vi "FPGA VI.vi"() -> ()   [LabVIEW 2026]
uses:
  <vilib>/rvi/Emulation/niFpgaGetClockAttributes.vi
  <vilib>/rvi/Emulation/niFpgaSctlEmulationGetInTimedLoop.vi
  <vilib>/rvi/Emulation/niFpgaEmulationReportErrorSimple.vi
  <vilib>/rvi/Emulation/niFpgaEmulationIsFPGAContextNoSignature.vi
  <vilib>/rvi/errors/niFpgaSetErrorForExecOnDevCompSimple.vi
  <vilib>/rvi/eio/common/nirviEmuReportErrorAndStop.vi
  <vilib>/rvi/DataTransferAndStorage/Container/Common/niFpgaContainerGetUniqueNameForEmu.vi
  <vilib>/rvi/FIFO/Fifo_Resource/nirvififoEmulationSetSize.vi
  <vilib>/rvi/FIFO/Fifo_Resource/nirviFifoEmulationQueueMgr.vi
  <instcachedir>/0/nirviFifoEmulationQueueMgr_E5CAEC123FF24DC58D834DCA3CDAA9B5.lvgen/nirviFifoEmulationQueueMgr_E5CAEC123FF24DC58D834DCA3CDAA9B5_002.vi
  <vilib>/Utility/error.llb/Clear Errors.vi
  <vilib>/rvi/FIFO/Fifo_Resource/nirvififoEmulationCreateLock.vi
  <vilib>/rvi/Emulation/niFpgaProcessEmulError.vi
  <vilib>/rvi/FIFO/Fifo_Resource/nirvififoEmulationObtainLock.vi
  <vilib>/rvi/FIFO/Fifo_Resource/nirvififoEmulationReleaseLock.vi
  <vilib>/rvi/occurrence/nirviWaitOnOccurrenceBase.vi
  <vilib>/rvi/errors/nirviReportUnexpectedCaseInternalError.vi
  <vilib>/rvi/errors/nirviReportUnexpectedCaseInternalError (U32).vi
  <vilib>/rvi/Emulation/niFpgaCriticalErrorInLSC.vi
  <vilib>/rvi/eio/common/nirviEmuTemplateMethod_errors.vi
  <vilib>/rvi/FIFO/Fifo_Resource/nirvififoEmulationDetermineInputValidOut.vi
  <vilib>/rvi/DataTransferAndStorage/Container/XNode/niFpgaContainer.xnode
  <vilib>/rvi/FIFO/Fifo_Resource/nirvififoEmulationRead.vi
  <vilib>/eio/EIONode/EIONode.xnode
  <vilib>/rvi/FIFO/Fifo_Resource/nirvififoEmulationWrite.vi
panel:
  out "appended array 3":bool[](array[boolean])
  out "appended array 2":bool[](array[boolean])
  out "appended array":bool[](array[boolean])
  in  "beep duration":i32=50
  in  "# of LED's lit at once":i16=11
  in  "activation threshold":u32=300
  out "Numeric":i32
  out "Time Since Last":u32=112
  in  "PWM Speaker Freq":u16[](array[numeric])=[432, 543, 754, 865, 1087]
  out "Iteratino Count":i32=5816678
  out "Time Left (ms)":i32
  in  "Random Index":i16
  out "Score":u16=718
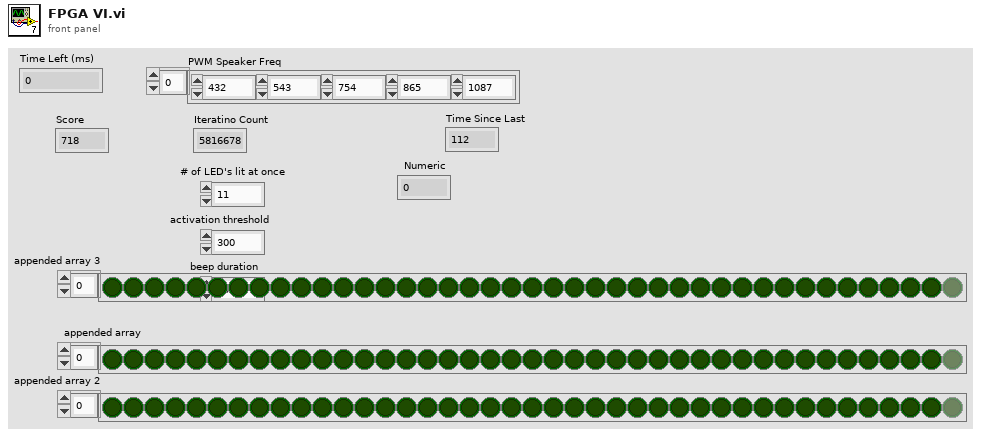
[diagram p1: front panel]
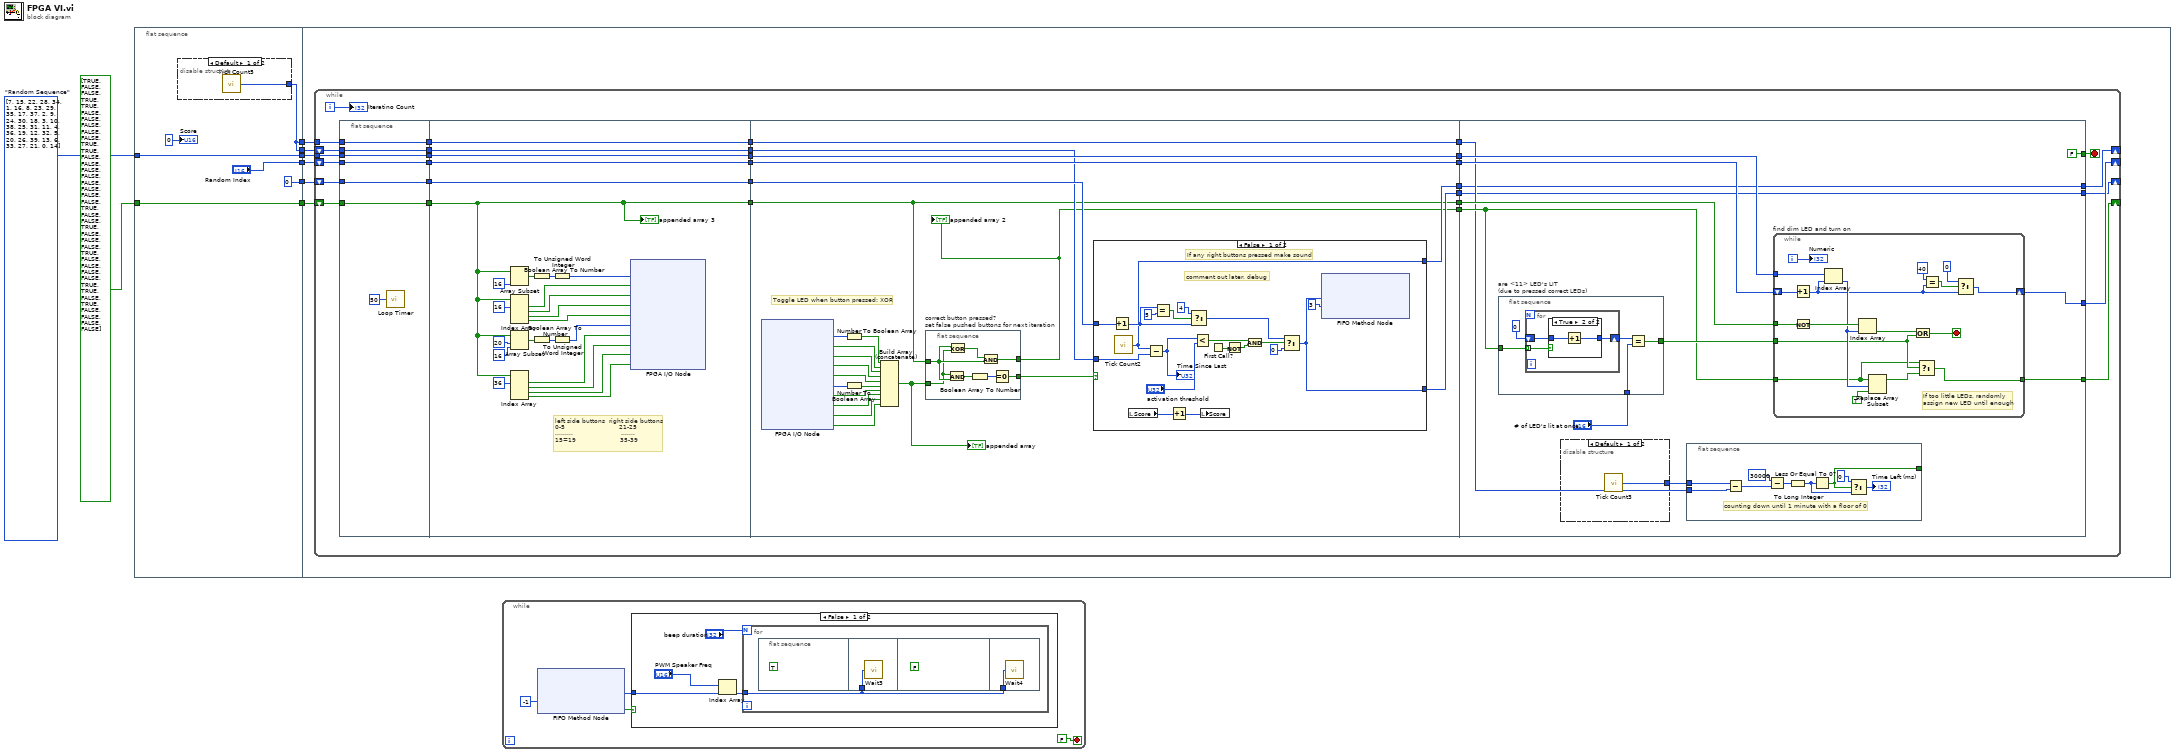
[diagram p0: block diagram]
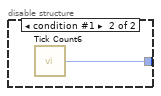
[diagram p3: hidden frame]
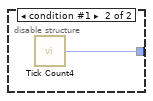
[diagram p5: hidden frame]
diagram:
  w2 = i16[] [7, 15, 22, 28, 34, 1, 16, 8, 23, 29, 35, 17, 37, 2, 9, 24, 30, 18, 3, 10, 38, 25, 31, 11, 4, 36, 19, 12, 32, 5, 20, 26, 39, 13, 6, 33, 27, 21, 0, 14]  # "Random Sequence"
  n1 = flat-sequence {
    tunnel: [w11] -> w8
    tunnel: [w10] -> w7
    tunnel: [w12] -> w6
    tunnel: ["Random Index"] -> w5
    tunnel: [u32 0 ("index")] -> w4
    tunnel: [w11] -> w3
    tunnel: w2 -> [w12]
    tunnel: bool[] [TRUE, FALSE, FALSE, TRUE, TRUE, FALSE, FALSE, FALSE, FALSE, FALSE, TRUE, TRUE, FALSE, FALSE, FALSE, FALSE, FALSE, FALSE, FALSE, FALSE, TRUE, FALSE, FALSE, TRUE, FALSE, FALSE, FALSE, TRUE, FALSE, FALSE, FALSE, FALSE, TRUE, TRUE, FALSE, TRUE, FALSE, FALSE, FALSE, FALSE] ("LEDs lit") -> [w10]
    tunnel: w8 -> [w19]
    tunnel: w7 -> [w22]
    tunnel: w6 -> [w21]
    tunnel: w5 -> [w20]
    tunnel: w4 -> [w18]
    tunnel: w3 -> [w17]
    frame #0 {
      n2 = disable-structure shown="Default" {
        disable-tunnel: [w15 w16] -> w11
        frame condition #0 (active) {
          n3 = call "Tick Count5"() -> ("Tick Count(mSec)"=w15:u32)
        }
        frame condition #1 {
          n4 = call "Tick Count6"() -> ("Tick Count(uSec)"=w16:u32)
        }
      }
      "Score" <- u16 0 ("Score 2")
    }
    frame #1 {
      n5 = while {
        shift-right: [w49] -> _
        shift-left: w22 -> [w52]
        tunnel: w21 -> [w45]
        shift-right: [w39] -> _
        shift-left: w20 -> [w41]
        tunnel: w19 -> [w35]
        shift-right: [w28] -> _
        shift-left: w18 -> [w30]
        shift-right: [w24] -> _
        shift-left: w17 -> [w25]
        i -> [w33]
        stop <- w34 stop-if-true
        n6 = flat-sequence {
          tunnel: [w59] -> w53
          tunnel: w52 -> [w59]
          tunnel: [w58] -> w46
          tunnel: w45 -> [w58]
          tunnel: [w57] -> w42
          tunnel: w41 -> [w57]
          tunnel: [w56] -> w36
          tunnel: w35 -> [w56]
          tunnel: [w55] -> w31
          tunnel: w30 -> [w55]
          tunnel: [w54] -> w26
          tunnel: w25 -> [w54]
          tunnel: w53 -> [w61]
          tunnel: [w61] -> w51
          tunnel: [w85] -> w47
          tunnel: w46 -> [w85]
          tunnel: [w84] -> w43
          tunnel: w42 -> [w84]
          tunnel: [w83] -> w37
          tunnel: w36 -> [w83]
          tunnel: [w82] -> w32
          tunnel: w31 -> [w82]
          tunnel: [w81] -> w27
          tunnel: w26 -> [w81]
          tunnel: w51 -> [w88]
          tunnel: [w86] -> w50
          tunnel: [w107] -> w48
          tunnel: w47 -> [w107]
          tunnel: [w106] -> w44
          tunnel: w43 -> [w106]
          tunnel: [w88] -> w40
          tunnel: [w105] -> w38
          tunnel: w37 -> [w105]
          tunnel: w32 -> [w104]
          tunnel: [w103] -> w29
          tunnel: w27 -> [w102]
          tunnel: [w101] -> w23
          tunnel: w50 -> [w147]
          tunnel: [w148] -> w49
          tunnel: w48 -> [w146]
          tunnel: w44 -> [w145]
          tunnel: w40 -> [w144]
          tunnel: [w143] -> w39
          tunnel: w38 -> [w142]
          tunnel: [FALSE] -> w34
          tunnel: w29 -> [w141]
          tunnel: [w141] -> w28
          tunnel: [w140] -> w24
          tunnel: w23 -> [w140]
          frame #0 {
            n7 = call "Loop Timer"("Count(uSec)"=u8 50 ("Count(Ticks)")) -> ()  [unwired: 1 out]
          }
          frame #1 {
            # "left side buttons  right side buttons\n0-5                           21-25\n.........                        .......  \n15=19                      35-39"
            n8 = Array Subset(array=w61, length=16) -> (w79:bool[])  [unwired: 1 in]
            n9 = Index Array(array=w61, index #1=16 ("index")) -> (element #1=w62:bool, element #2=w65:bool, element #3=w64:bool, element #4=w63:bool)  [unwired: 3 in]
            n10 = Array Subset(array=w61, index=20, length=16) -> (w74:bool[])
            n11 = Index Array(array=w61, index #1=36 ("index")) -> (element #1=w70:bool, element #2=w68:bool, element #3=w67:bool, element #4=w66:bool)  [unwired: 3 in]
            n12 = Boolean Array To Number(Boolean array=w79) -> (number=w78:u16)
            n13 = Boolean Array To Number(Boolean array=w74) -> (number=w75:u16)
            n14 = To Unsigned Word Integer(number=w78) -> (unsigned 16bit integer=w77:u16)
            n15 = To Unsigned Word Integer(number=w75) -> (unsigned 16bit integer=w69:u16)
            n16 = xnode "FPGA I/O Node"("Bank-01/DO15:0"=w77, "Bank-03/DO0"=w62, "Bank-03/DO1"=w65, "Bank-03/DO2"=w64, "Bank-03/DO3"=w63, "Bank-02/DO15:0"=w69, "Bank-03/DO4"=w70, "Bank-03/DO5"=w68, "Bank-03/DO6"=w67, "Bank-03/DO7"=w66) -> ()  [unwired: 10 in, 10 out]
            "appended array 3" <- w61
          }
          frame #2 {
            # "Toggle LED when button pressed: XOR"
            n17 = xnode "FPGA I/O Node"() -> ("Bank-01/DI15:0"=w108:u16, "Bank-03/DI0"=w90:bool, "Bank-03/DI1"=w99:bool, "Bank-03/DI2"=w98:bool, "Bank-03/DI3"=w97:bool, "Bank-02/DI15:0"=w92:u16, "Bank-03/DI4"=w96:bool, "Bank-03/DI5"=w95:bool, "Bank-03/DI6"=w94:bool, "Bank-03/DI7"=w93:bool)  [unwired: 10 in, 10 out]
            n18 = Number To Boolean Array(number=w108) -> (Boolean array=w100:bool[])
            n19 = Number To Boolean Array(number=w92) -> (Boolean array=w91:bool[])
            n20 = Build Array (concatenate)(w100, w90, w99, w98, w97, w91, w96, w95, w94, w93) -> (w87:bool[])
            "appended array" <- w87
            n21 = flat-sequence "correct button pressed?\nset false pushed buttons for next iteration" {
              tunnel: [w114] -> w86
              tunnel: [w111] -> w89
              tunnel: w88 -> [w110]
              tunnel: w87 -> [w109]
              frame #0 {
                n22 = And(x=w109, y=w110) -> (x .and. y?=w113:bool[])
                n23 = Exclusive Or(1:w109, 2:w110) -> (0:w115:bool[])
                n24 = Boolean Array To Number(Boolean array=w113) -> (number=w112:u64)
                n25 = And(x=w115, y=w110) -> (x .and. y?=w114:bool[])
                n26 = Equal To 0?(x=w112) -> (x = 0?=w111:bool)
              }
            }
            n27 = case shown="False" w89 {
              tunnel: w104 -> [w125 w136]
              tunnel: [w116 w136] -> w103
              tunnel: w102 -> [w118 w135]
              tunnel: [w117 w135] -> w101
              frame False {
                # "comment out later, debug"
                # "If any right buttons pressed make sound"
                n28 = Increment(x=w125) -> (x+1=w128:u32)
                n29 = call "Tick Count2"() -> ("Tick Count(mSec)"=w117:u32)
                n30 = local read "Score"() -> (w134:u16)
                n31 = Subtract(x=w117, y=w118) -> (x-y=w119:u32)
                "Time Since Last" <- w119
                n32 = Equal?(x=w128, y=u32 5) -> (x = y?=w130:bool)
                n33 = Increment(x=w134) -> (x+1=w133:u16)
                n34 = Select(t=u32 4, s=w130, f=w128) -> (s? t:f=w126:u32)
                n35 = Less?(x=w119, y="activation threshold") -> (x < y?=w123:bool)
                n36 = local write "Score"(w133) -> ()
                n37 = First Call?() -> (First Call?: T/F=w121:bool)
                n38 = Not(x=w121) -> (.not. x?=w124:bool)
                n39 = And(x=w123, y=w124) -> (x .and. y?=w122:bool)
                n40 = Select(t=w126, s=w122, f=u32 0) -> (s? t:f=w116:u32)
                n41 = xnode ("FIFO Method Node")("Element"=w116, "Timeout"=3) -> ()  [unwired: 1 in, 2 out]
              }
              frame True {
              }
            }
            "appended array 2" <- w86
          }
          frame #3 {
            n42 = flat-sequence "are <11> LED's LIT\n(due to pressed correct LEDs)" {
              tunnel: [w165] -> w149
              tunnel: w147 -> [w164]
              tunnel: "# of LED's lit at once" -> [w161]
              frame #0 {
                n43 = for {
                  tunnel: w164 -> [w166] mode=indexing
                  shift-right: [w168] -> w163
                  shift-left: i16 0 -> [w167]
                  n44 = case shown="True" w166 {
                    tunnel: [w169 w171] -> w168
                    tunnel: w167 -> [w169 w170]
                    frame False {
                    }
                    frame True {
                      n45 = Increment(x=w170) -> (x+1=w171:i16)
                    }
                  }
                }
                n46 = Equal?(x=w163, y=w161) -> (x = y?=w165:bool)
              }
            }
            n47 = disable-structure shown="Default" {
              disable-tunnel: [w150 w151] -> w138
              frame condition #0 (active) {
                n48 = call "Tick Count3"() -> ("Tick Count(mSec)"=w150:u32)
              }
              frame condition #1 {
                n49 = call "Tick Count4"() -> ("Tick Count(uSec)"=w151:u32)
              }
            }
            n50 = flat-sequence {
              tunnel: w142 -> [w160]
              tunnel: [w156] -> _
              tunnel: w138 -> [w152]
              frame #0 {
                # "counting down until 1 minute with a floor of 0"
                n51 = Subtract(x=w152, y=w160) -> (x-y=w159:u32)
                n52 = Subtract(x=u32 30000, y=w159) -> (x-y=w157:u32)
                n53 = To Long Integer(number=w157) -> (32bit integer=w155:i32)
                n54 = Less Or Equal To 0?(x=w155) -> (x <= 0?=w156:bool)
                n55 = Select(t=0, s=w156, f=w155) -> (s? t:f=→"Time Left (ms)":i32)
              }
            }
            n56 = while "find dim LED and turn on" {
              tunnel: w149 -> [w178]
              tunnel: w146 -> [w181]
              tunnel: w144 -> [w177]
              shift-right: [w187] -> w143
              shift-left: w145 -> [w185]
              tunnel: w147 -> [w174]
              tunnel: [w175] -> w148
              i -> [w173]
              stop <- w179 stop-if-true
              # "If too little LEDs, randomly\nassign new LED until enough"
              n57 = Increment(x=w185) -> (x+1=w172:i16)
              n58 = Not(x=w177) -> (.not. x?=w184:bool[])
              n59 = Index Array(array=w181, index=w172) -> (element=w180:i16)
              n60 = Index Array(array=w184, index=w180) -> (element=w182:bool)
              n61 = Replace Array Subset(array=w174, new element=TRUE ("new element/subarray"), index=w180) -> (w176:bool[])
              n62 = Or(x=w182, y=w178) -> (x .or. y?=w179:bool)
              n63 = Select(t=w174, s=w178, f=w176) -> (s? t:f=w175:bool[])
              n64 = Equal?(x=i16 40 ("y"), y=w172) -> (x = y?=w189:bool)
              n65 = Select(t=i16 0, s=w189, f=w172) -> (s? t:f=w187:i16)
              "Numeric" <- w173
            }
          }
        }
        "Iteratino Count" <- w33
      }
    }
  }
  n66 = while {
    stop <- FALSE ("stop") stop-if-true
    n67 = xnode ("FIFO Method Node")("Timeout"=-1) -> ("Element"=w192:u8, "Timed Out?"=w190:bool)  [unwired: 1 in, 1 out]
    n68 = case shown="False" w190 {
      tunnel: w192 -> [w196 _]
      frame False {
        n69 = Index Array(array="PWM Speaker Freq", index=w196) -> (element=w197:u16)
        n70 = for {
          N: "beep duration" -> [_]
          tunnel: w197 -> [w198]
          n71 = flat-sequence {
            tunnel: w198 -> [w199]
            tunnel: w198 -> [w200]
            frame #0 {
              (unwired) TRUE ("Mod1/DO0")
            }
            frame #1 {
              n72 = call "Wait3"("Count(uSec)"=w199) -> ()  [unwired: 1 out]
            }
            frame #2 {
              (unwired) FALSE ("Mod1/DO0")
            }
            frame #3 {
              n73 = call "Wait4"("Count(uSec)"=w200) -> ()  [unwired: 1 out]
            }
          }
        }
      }
      frame True {
      }
    }
  }
